vi "Execute SQL.vi"(8 "error in":errorcluster, 10 "SQL":string, 11 "Data.PG":refnum<class "Data.PGSQL.lvclass">) -> (0 "error out":errorcluster, 2 "Result":string[][](array[string]), 3 "Data.PG out":refnum<class "Data.PGSQL.lvclass">)   [LabVIEW 2013, in "Data.PGSQL.lvclass"]
uses:
  Data.PGSQL.lvclass
  PostgreSQL Library/Connection/PQ Connection.lvclass
  Data.PGSQL.lvclass/Data.PGSQL.ctl
  PostgreSQL Library/Result/PQ Result.lvclass/PQ Result.ctl
  PostgreSQL Library/Connection/Execute Command (2D string results).vi
  PostgreSQL Library/Result/Clear.vi
  PostgreSQL Library/Connection/Execute Command (Result).vi
  PostgreSQL Library/Result/Get all results as 2D strings array.vi
  PostgreSQL Library/Connection/Execute (Return first result with rows).vi
  PostgreSQL Library/Connection/Single Command with parameters.vi
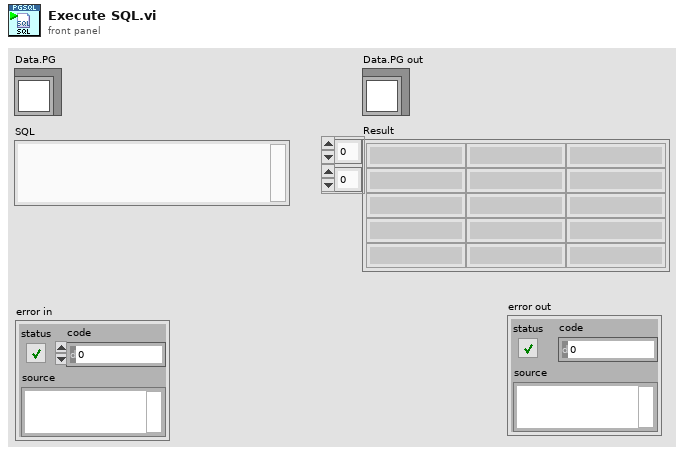
[diagram p1: front panel]
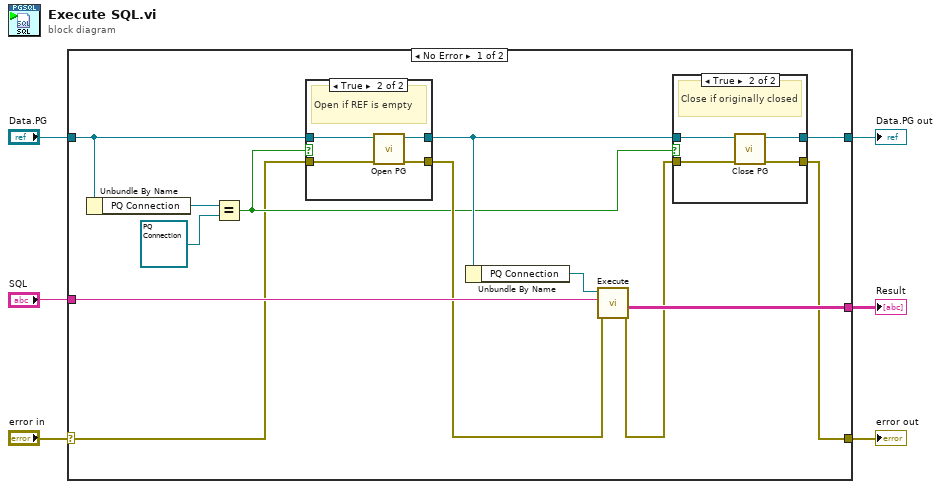
[diagram p0: block diagram]
diagram:
  n1 = case shown="No Error" "error in" {
    selector: "error in" -> [w7 w32]
    tunnel: [w19 _] -> w6
    tunnel: "SQL" -> [w18 _]
    tunnel: [w14 w32] -> w4
    tunnel: [w13 w33] -> w3
    tunnel: "Data.PG" -> [w9 w33]
    frame No Error {
      n2 = Unbundle By Name(w9) -> ("PQ Connection"=w11:refnum<class "PQ Connection.lvclass">)
      n3 = Equal?(x=w11, y=refnum<class "PQ Connection.lvclass"> refnum ("PQ Connection")) -> (x = y?=w8:bool)
      n4 = case shown="True" w8 {
        tunnel: w9 -> [w20 w23]
        tunnel: [w20 w25] -> w16
        tunnel: [w21 w24] -> w17
        tunnel: w7 -> [w21 w22]
        frame False {
        }
        frame True {
          # "Open if REF is empty"
          n5 = call-dynamic "Open PG.vi"("error in (no error)"=w22, "Data.PG in"=w23) -> ("error out"=w24:errorcluster, "Data.PG out"=w25:refnum<class "Data.PGSQL.lvclass">)  [unwired: 8 in]
        }
      }
      n6 = Unbundle By Name(w16) -> ("PQ Connection"=w12:refnum<class "PQ Connection.lvclass">)
      n7 = call-poly "Execute.vi"("error in (no error)"=w17, "SQL"=w18, "PQ Connection in"=w12) -> ("error out"=w15:errorcluster, "Result"=w19:string[][])  [unwired: 5 in, 2 out]
      n8 = case shown="True" w8 {
        tunnel: w16 -> [w26 w31]
        tunnel: w15 -> [w27 w30]
        tunnel: [w27 w29] -> w14
        tunnel: [w26 w28] -> w13
        frame False {
          # "Do not close if closed wasn't before"
        }
        frame True {
          # "Close if originally closed"
          n9 = call-dynamic "Close PG.vi"("error in (no error)"=w30, "Data.PG in"=w31) -> ("error out"=w29:errorcluster, "Data.PG out"=w28:refnum<class "Data.PGSQL.lvclass">)  [unwired: 8 in]
        }
      }
    }
    frame Error {
    }
  }
  "Result" <- w6
  "error out" <- w4
  "Data.PG out" <- w3
